vi "计算扇区起点终点.vi"(10 "角度":dbl, 11 "Fitted Circle (Find Circular Edge 1)":T2 {"Average SNR (dB)" format="%.2f"; "Average Strength" format="%.2f"; "Roundness (Real-World)" format="%.2f"; "Radius (Real-World)" format="%.2f"; "Center (Real-World)"."Y" format="%.2f"; "Center (Real-World)"."X" format="%.2f"; "Radius (Pixels)" format="%.2f"; "Center (Pixels)"."Y" format="%.2f"; "Center (Pixels)"."X" format="%.2f"}) -> (0 "EndPos":cluster{"dx":dbl, "dy":dbl}, 1 "StartPos":cluster{"X":sgl, "Y":sgl}, 2 "y out":dbl caption="y输出", 3 "X":dbl caption="x输出", 4 "输出簇":T1 {"Start X" scale=0.0..1024.0; "End X" scale=0.0..1024.0})   [LabVIEW 2017]
uses:
  <vilib>/Analysis/coordinate.llb/2D Cartesian Coordinate Shift (Scalar).vi
  <vilib>/Analysis/NI_AALPro.lvlib
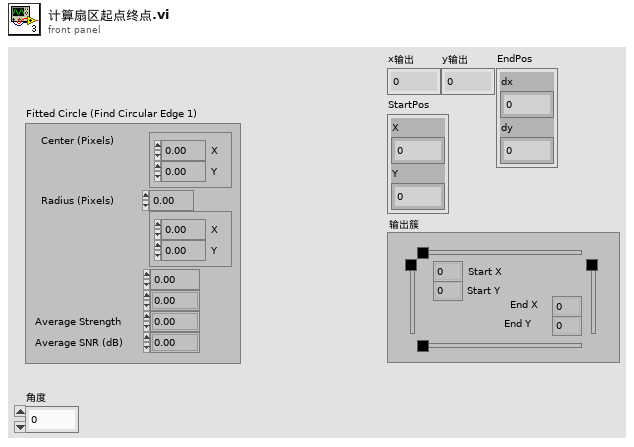
[diagram p1: front panel]
types:
  T1 = typedef "IMAQ Line" = cluster{"Start X":i32, "Start Y":i32, "End X":i32, "End Y":i32}
  T2 = cluster{"Center (Pixels)":cluster{"X":sgl, "Y":sgl}, "Radius (Pixels)":dbl, "Center (Real-World)":cluster{"X":sgl, "Y":sgl}, "Radius (Real-World)":dbl, "Roundness (Real-World)":dbl, "Average Strength":dbl, "Average SNR (dB)":dbl}
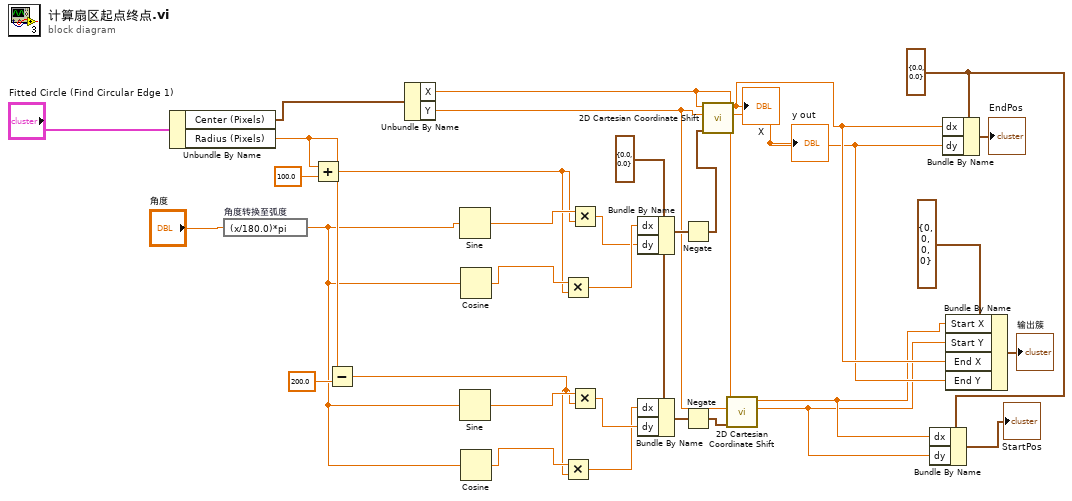
[diagram p0: block diagram]
diagram:
  w2 = cluster{"dx":dbl, "dy":dbl} {"dx"=0.0, "dy"=0.0} ("shift")
  w9 = cluster{"dx":dbl, "dy":dbl} {"dx"=0.0, "dy"=0.0} ("shift")
  n1 = Unbundle By Name("Fitted Circle (Find Circular Edge 1)") -> ("Center (Pixels)"=w31:cluster{"X":sgl, "Y":sgl}, "Radius (Pixels)"=w16:dbl)
  n2 = expression code="(x/180.0)*pi" "角度转换至弧度"("角度") -> (w11:dbl)
  n3 = Add(x=w16, y=100.0) -> (x+y=w22:dbl)
  n4 = Subtract(x=w16, y=200.0) -> (x-y=w10:dbl)
  n5 = Unbundle By Name(w31) -> ("X"=w6:sgl, "Y"=w5:sgl)
  n6 = Sine(x=w11) -> (sin(x)=w29:dbl)
  n7 = Sine(x=w11) -> (sin(x)=w12:dbl)
  n8 = Cosine(x=w11) -> (cos(x)=w28:dbl)
  n9 = Cosine(x=w11) -> (cos(x)=w13:dbl)
  n10 = Multiply(x=w28, y=w22) -> (x*y=w27:dbl)
  n11 = Multiply(x=w13, y=w10) -> (x*y=w14:dbl)
  n12 = Multiply(x=w29, y=w22) -> (x*y=w26:dbl)
  n13 = Multiply(x=w12, y=w10) -> (x*y=w15:dbl)
  n14 = Bundle By Name(cluster=w9, "dx"=w27, "dy"=w26) -> (w25:cluster{"dx":dbl, "dy":dbl})
  n15 = Bundle By Name(cluster=w9, "dx"=w14, "dy"=w15) -> (w8:cluster{"dx":dbl, "dy":dbl})
  n16 = Negate(x=w25) -> (-x=w24:cluster{"dx":dbl, "dy":dbl})
  n17 = Negate(x=w8) -> (-x=w7:cluster{"dx":dbl, "dy":dbl})
  n18 = call-poly <vilib>:"2D Cartesian Coordinate Shift.vi"("shift"=w24, "y"=w5, "x"=w6) -> ("y out"=w19:dbl, "x out"=w20:dbl)  [unwired: 6 in, 1 out]
  "X" <- w20
  "y out" <- w19
  n19 = call-poly <vilib>:"2D Cartesian Coordinate Shift.vi"("shift"=w7, "y"=w5, "x"=w6) -> ("y out"=w3:dbl, "x out"=w4:dbl)  [unwired: 6 in, 1 out]
  n20 = Bundle By Name(cluster=w2, "dx"=w4, "dy"=w3) -> (→"StartPos":cluster{"dx":dbl, "dy":dbl})
  n21 = Bundle By Name(cluster=w2, "dx"=w20, "dy"=w19) -> (→"EndPos":cluster{"dx":dbl, "dy":dbl})
  n22 = Bundle By Name(cluster=T1 {"Start X"=0, "Start Y"=0, "End X"=0, "End Y"=0} ("Line"), "Start X"=w4, "Start Y"=w3, "End X"=w20, "End Y"=w19) -> (→"输出簇":T1)
